vi "OpenHDF5.vi"(8 "error in (no error)":errorcluster, 9 "appended path":path, 10 "Save Analog Signals":bool=TRUE, 11 "Photodiode in":refnum<class "Photodiode.lvclass">) -> (0 "error out":errorcluster, 3 "Photodiode out":refnum<class "Photodiode.lvclass">)   [LabVIEW 2016, in "Photodiode.lvclass"]
uses:
  Photodiode.lvclass
  Photodiode.lvclass/Photodiode.ctl
  private/HDF5Tools32/LabView/Create Dataset 2D Double.vi
  private/HDF5Tools32/LabView/HDF5Tools.lvlib
panel:
  in  "Rate":dbl=10000.0 caption="Sample Rate (Hz)" format="%0.2f"
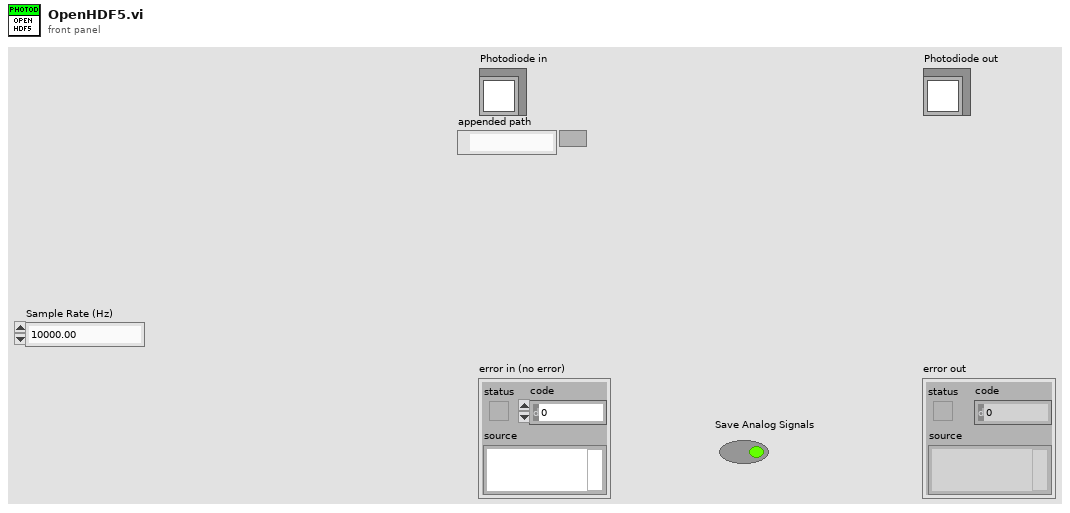
[diagram p1: front panel]
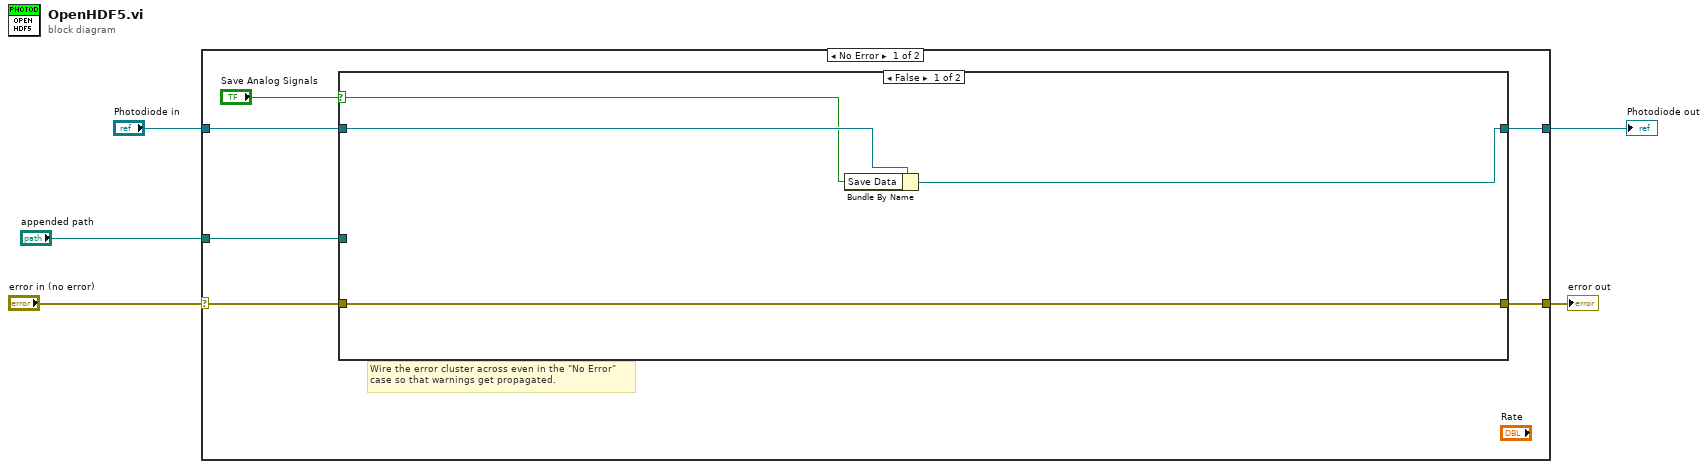
[diagram p0: block diagram]
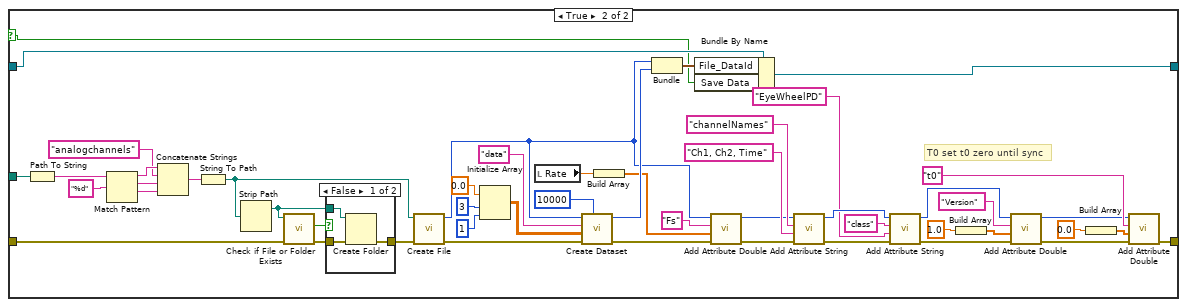
[diagram p2: hidden frame]
diagram:
  n1 = case shown="No Error" "error in (no error)" {
    selector: "error in (no error)" -> [w10 w71]
    tunnel: [w9 w71] -> w4
    tunnel: [w6 w70] -> w2
    tunnel: "Photodiode in" -> [w7 w70]
    tunnel: "appended path" -> [w8 _]
    frame No Error {
      # "Wire the error cluster across even in the \"No Error\"\ncase so that warnings get propagated."
      n2 = case shown="False" "Save Analog Signals" {
        selector: "Save Analog Signals" -> [w12 w16]
        tunnel: w8 -> [_ w65]
        tunnel: [w15 w22] -> w9
        tunnel: w10 -> [w15 w20]
        tunnel: w7 -> [w14 w19]
        tunnel: [w13 w18] -> w6
        frame False {
          n3 = Bundle By Name(cluster=w14, "Save Data"=w12) -> (w13:refnum<class "Photodiode.lvclass">)
        }
        frame True {
          # "T0 set t0 zero until sync"
          n4 = Path To String(path=w65) -> (string=w35:string)
          n5 = Match Pattern(string=w35, regular expression="%d") -> (before substring=w33:string, match substring=w31:string, after substring=w30:string)  [unwired: 1 in, 1 out]
          n6 = Concatenate Strings(w33, "analogchannels" ("string"), w31, w30) -> (w29:string)
          n7 = String To Path(string=w29) -> (path=w21:path)
          n8 = Strip Path(path=w21) -> (stripped path=w28:path)  [unwired: 1 out]
          n9 = call <vilib>:"Check if File or Folder Exists.vi"("error in (no error)"=w20, "path"=w28) -> ("error out"=w26:errorcluster, "file or folder exists?"=w27:bool)  [unwired: 7 in, 1 out]
          n10 = case shown="False" w27 {
            tunnel: w28 -> [w68 _]
            tunnel: w26 -> [w67 w69]
            tunnel: [w66 w69] -> w40
            frame False {
              n11 = Create Folder(path (use dialog)=w68, error in=w67) -> (error out=w66:errorcluster)  [unwired: 1 in, 2 out]
            }
            frame True {
            }
          }
          n12 = call "Create File.vi"("Error in"=w40, "File Name"=w21) -> ("Error out"=w64:errorcluster, "file_id"=w55:i32)  [unwired: 6 in]
          n13 = Initialize Array(0.0, 3 ("dimension size"), 1 ("dimension size")) -> (w59:dbl[][])
          n14 = local read "Rate"() -> (w25:dbl)
          n15 = call-poly "Create Dataset.vi"("Chunk size"=10000, "error in (no error)"=w64, "Datatype"=w59, "Dataset name"="data", "Location id in"=w55) -> ("error out"=w54:errorcluster, "Dataset id"=w58:i32)  [unwired: 5 in]
          n16 = Build Array(w25) -> (w24:dbl[])
          n17 = Bundle("file_id"=w55, "Dataset id"=w58) -> (w17:cluster{"file_id":i32, "Dataset id":i32})  [unwired: 1 in]
          n18 = Bundle By Name(cluster=w19, "File_DataId"=w17, "Save Data"=w16) -> (w18:refnum<class "Photodiode.lvclass">)
          n19 = call "Add Attribute Double.vi"("error in (no error)"=w54, "data"=w24, "Attribute name"="Fs", "loc_id"=w55) -> ("error out"=w36:errorcluster, "loc_id_out"=w37:i32)  [unwired: 6 in]
          n20 = call "Add Attribute String.vi"("error in (no error)"=w36, "Attribute data"="Ch1, Ch2, Time", "Attribute name"="channelNames", "loc_id"=w37) -> ("error out"=w51:errorcluster, "loc_id_out"=w53:i32)  [unwired: 6 in]
          n21 = call "Add Attribute String.vi"("error in (no error)"=w51, "Attribute data"="EyeWheelPD", "Attribute name"="class", "loc_id"=w53) -> ("error out"=w48:errorcluster, "loc_id_out"=w46:i32)  [unwired: 6 in]
          n22 = Build Array(1.0) -> (w47:dbl[])
          n23 = call "Add Attribute Double.vi"("error in (no error)"=w48, "data"=w47, "Attribute name"="Version", "loc_id"=w46) -> ("error out"=w43:errorcluster, "loc_id_out"=w42:i32)  [unwired: 6 in]
          n24 = Build Array(0.0 ("element")) -> (w44:dbl[])
          n25 = call "Add Attribute Double.vi"("error in (no error)"=w43, "data"=w44, "Attribute name"="t0", "loc_id"=w42) -> ("error out"=w22:errorcluster)  [unwired: 6 in, 1 out]
        }
      }
    }
    frame Error {
    }
  }
  "error out" <- w4
  "Photodiode out" <- w2
